vi "Read password.vi"(8 "error in (no error)":errorcluster, 11 "Generic Client in":refnum<class "Generic Client.lvclass">) -> (0 "error out":errorcluster, 2 "password":string, 3 "Generic Client out":refnum<class "Generic Client.lvclass">)   [LabVIEW 2020, in "NI_SSH.lvlib" / "Generic Client.lvclass"]
uses:
  <vilib>/net/SSH/Client/Generic/Generic Client.lvclass
  <vilib>/net/SSH/Client/Generic/Generic Client.lvclass/Generic Client.ctl
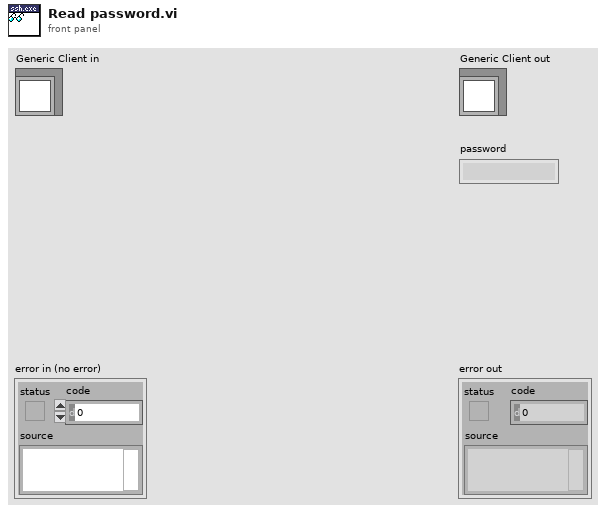
[diagram p1: front panel]
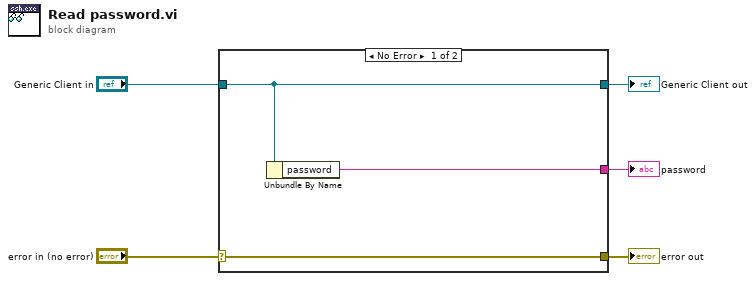
[diagram p0: block diagram]
diagram:
  n1 = case shown="No Error" "error in (no error)" {
    selector: "error in (no error)" -> [w8 w9]
    tunnel: [w8 w9] -> w4
    tunnel: [w7 w10] -> w2
    tunnel: "Generic Client in" -> [w7 w10]
    tunnel: [w6 _] -> w1
    frame No Error {
      n2 = Unbundle By Name(w7) -> ("password"=w6:string)
    }
    frame Error {
    }
  }
  "error out" <- w4
  "Generic Client out" <- w2
  "password" <- w1
